vi "Read Sorted scan parameters.vi"(8 "error in (no error)":errorcluster, 11 "SweepControl in":refnum<class "SweepControl.lvclass">) -> (0 "error out":errorcluster, 2 "Sorted scan parameters":cluster{T1}[](array[cluster])=[{[{"Start"=0.14, "End"=-0.060000000000000005, "Step"=-0.060000000000000005, "Rate"=0.0, "wait (ms/mK)"=10000, "Address"="Dev2/ao0", "channel"=1}]}, {[{"Start"=0.14, "End"=-0.060000000000000005, "Step"=-0.060000000000000005, "Rate"=0.0, "wait (ms/mK)"=10000, "Address"="Dev2/ao0", "channel"=1}]}, {[{"Start"=0.14, "End"=-0.060000000000000005, "Step"=-0.060000000000000005, "Rate"=0.0, "wait (ms/mK)"=10000, "Address"="Dev2/ao0", "channel"=1}, {"Start"=0.14, "End"=-0.060000000000000005, "Step"=-0.060000000000000005, "Rate"=0.0, "wait (ms/mK)"=10000, "Address"="Dev2/ao0", "channel"=1}]}] {"?"."Rate" format="%.2f"; "?"."Step" format="%#_6p"; "?"."End" format="%#_6p"; "?"."Start" format="%#_6p"}, 3 "SweepControl out":refnum<class "SweepControl.lvclass">)   [LabVIEW 2020, in "SweepControl.lvclass"]
uses:
  SweepControl.lvclass
  Typedefs/ScanParamters.ctl
  Typedefs/Cluster - ScanParamters.ctl
  SweepControl.lvclass/SweepControl.ctl
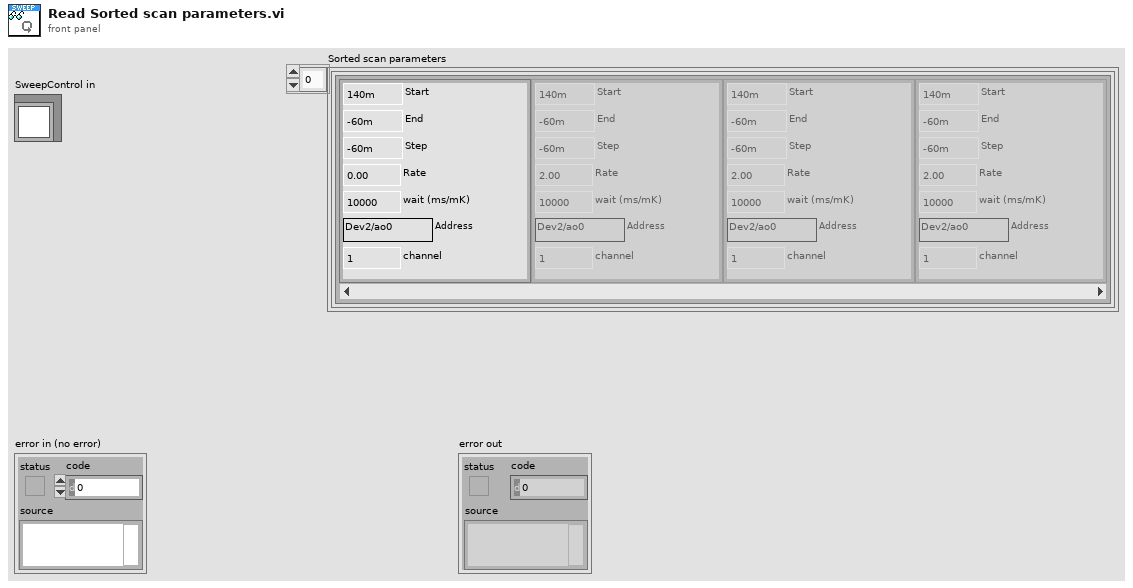
[diagram p1: front panel]
types:
  T1 = typedef "SweepControl.lvclass/ScanParamters.ctl" = T2[]
  T2 = typedef "SweepControl.lvclass/Cluster - ScanParamters.ctl" = cluster{"Start":dbl, "End":dbl, "Step":dbl, "Rate":dbl, "wait (ms/mK)":u32, "Address":string, "channel":i32}
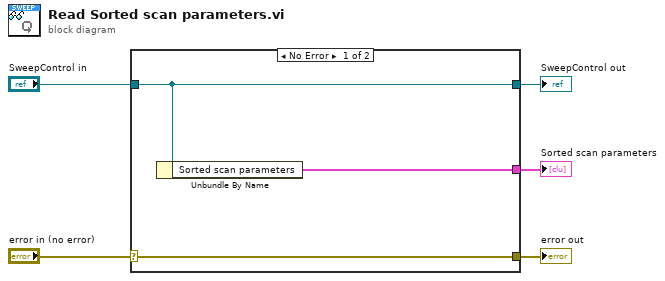
[diagram p0: block diagram]
diagram:
  n1 = case shown="No Error" "error in (no error)" {
    selector: "error in (no error)" -> [w8 w9]
    tunnel: [w8 w9] -> w4
    tunnel: [w7 w10] -> w2
    tunnel: "SweepControl in" -> [w7 w10]
    tunnel: [w6 _] -> w1
    frame No Error {
      n2 = Unbundle By Name(w7) -> ("Sorted scan parameters"=w6:cluster{T1}[])
    }
    frame Error {
    }
  }
  "error out" <- w4
  "SweepControl out" <- w2
  "Sorted scan parameters" <- w1
